vi "Fetch Rooms List.vi"(0 "File Data Manager in":refnum<class "File Data Manager.lvclass">, 11 "error in (no error)":errorcluster) -> (4 "File Data Manager out":refnum<class "File Data Manager.lvclass">, 6 "Room No":string[](array[string]), 15 "error out":errorcluster)   [LabVIEW 2023, in "File Data Manager.lvlib" / "File Data Manager.lvclass"]
uses:
  File Data Manager.lvclass
  File Data Manager.lvclass/File Data Manager.ctl
  Central Data Manager/Central Data Manager/Central Data Manager.lvclass
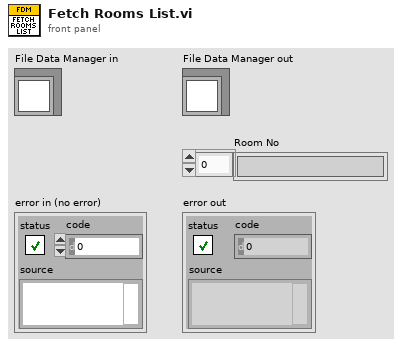
[diagram p1: front panel]
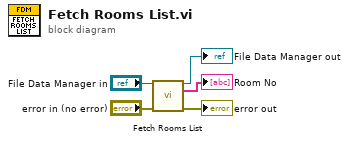
[diagram p0: block diagram]
diagram:
  n1 = call-parent "Fetch Rooms List.vi"("Central Data Manager in"="File Data Manager in", "error in (no error)"="error in (no error)") -> ("Central Data Manager out"=→"File Data Manager out":refnum<class "File Data Manager.lvclass">, "Room No"=→"Room No":string[], "error out"=→"error out":errorcluster)  [unwired: 11 in]
